vi "Reader.vi"() -> ()   [LabVIEW 2017]
uses:
  <vilib>/Instr/_visa.llb/VISA Configure Serial Port (Instr).vi
  <vilib>/picture/3D Picture Control/NI_3D Picture Control.lvlib
  <userlib>/_MGI/Numeric/Coercion/MGI Degrees to Radians/MGI Degrees to Radians DBL.vi
panel:
  out "result":i32
  out "sqrt(x)":dbl format="%#.1f"
  out "Samples (float)":dbl
  out "Gyro":cluster{"Pos X":dbl, "Pos Y":dbl, "Pos Z":dbl} {"Pos Z" format="%#.1f"; "Pos Y" format="%#.1f"; "Pos X" format="%#.1f"}
  out "Acc":cluster{"Pos X":dbl, "Pos Y":dbl, "Pos Z":dbl} {"Pos Z" format="%#.1f"; "Pos Y" format="%#.1f"; "Pos X" format="%#.1f"}
  out "Both":cluster{"Pos X":dbl, "Pos Y":dbl, "Pos Z":dbl} {"Pos Z" format="%#.1f"; "Pos Y" format="%#.1f"; "Pos X" format="%#.1f"}
  out "Pos":cluster{"Pos X":dbl, "Pos Y":dbl, "Pos Z":dbl} {"Pos Z" format="%#.1f"; "Pos Y" format="%#.1f"; "Pos X" format="%#.1f"}
  in  "Reading type":enum16{"ER_READ", "ER_BUF", "None"}(ring)
  in  "Fs reading":dbl=50.0 format="%#_13g"
  out "Acc Z":i16 caption="Z"
  out "Acc Y":i16 caption="Y"
  out "Acc X":i16 caption="X"
  out "Gyro Z":i16 caption="Z"
  out "Gyro Y":i16 caption="Y"
  out "Gyro X":i16 caption="X"
  out "Read":refnum<vi>(3d-picture)
  out "Samples (Int)":i32
  in  "Gyro LSB":dbl=131.0 format="%#_13g"
  out "error out":errorcluster
  out "Not recognized command":string
  in  "VISA resource name":refnum<visa-resource-name>="COM3"
  out "Gyro":refnum<vi>(3d-picture)
  out "Acc":refnum<vi>(3d-picture)
  in  "Gyro %":dbl=0.9 min=0.0 max=1.0 step=0.01
  out "Both":refnum<vi>(3d-picture)
  # "Comm setting"
  # "Positions"
  # "Reading"
  # "values"
  # "Acc"
  # "Gyro"
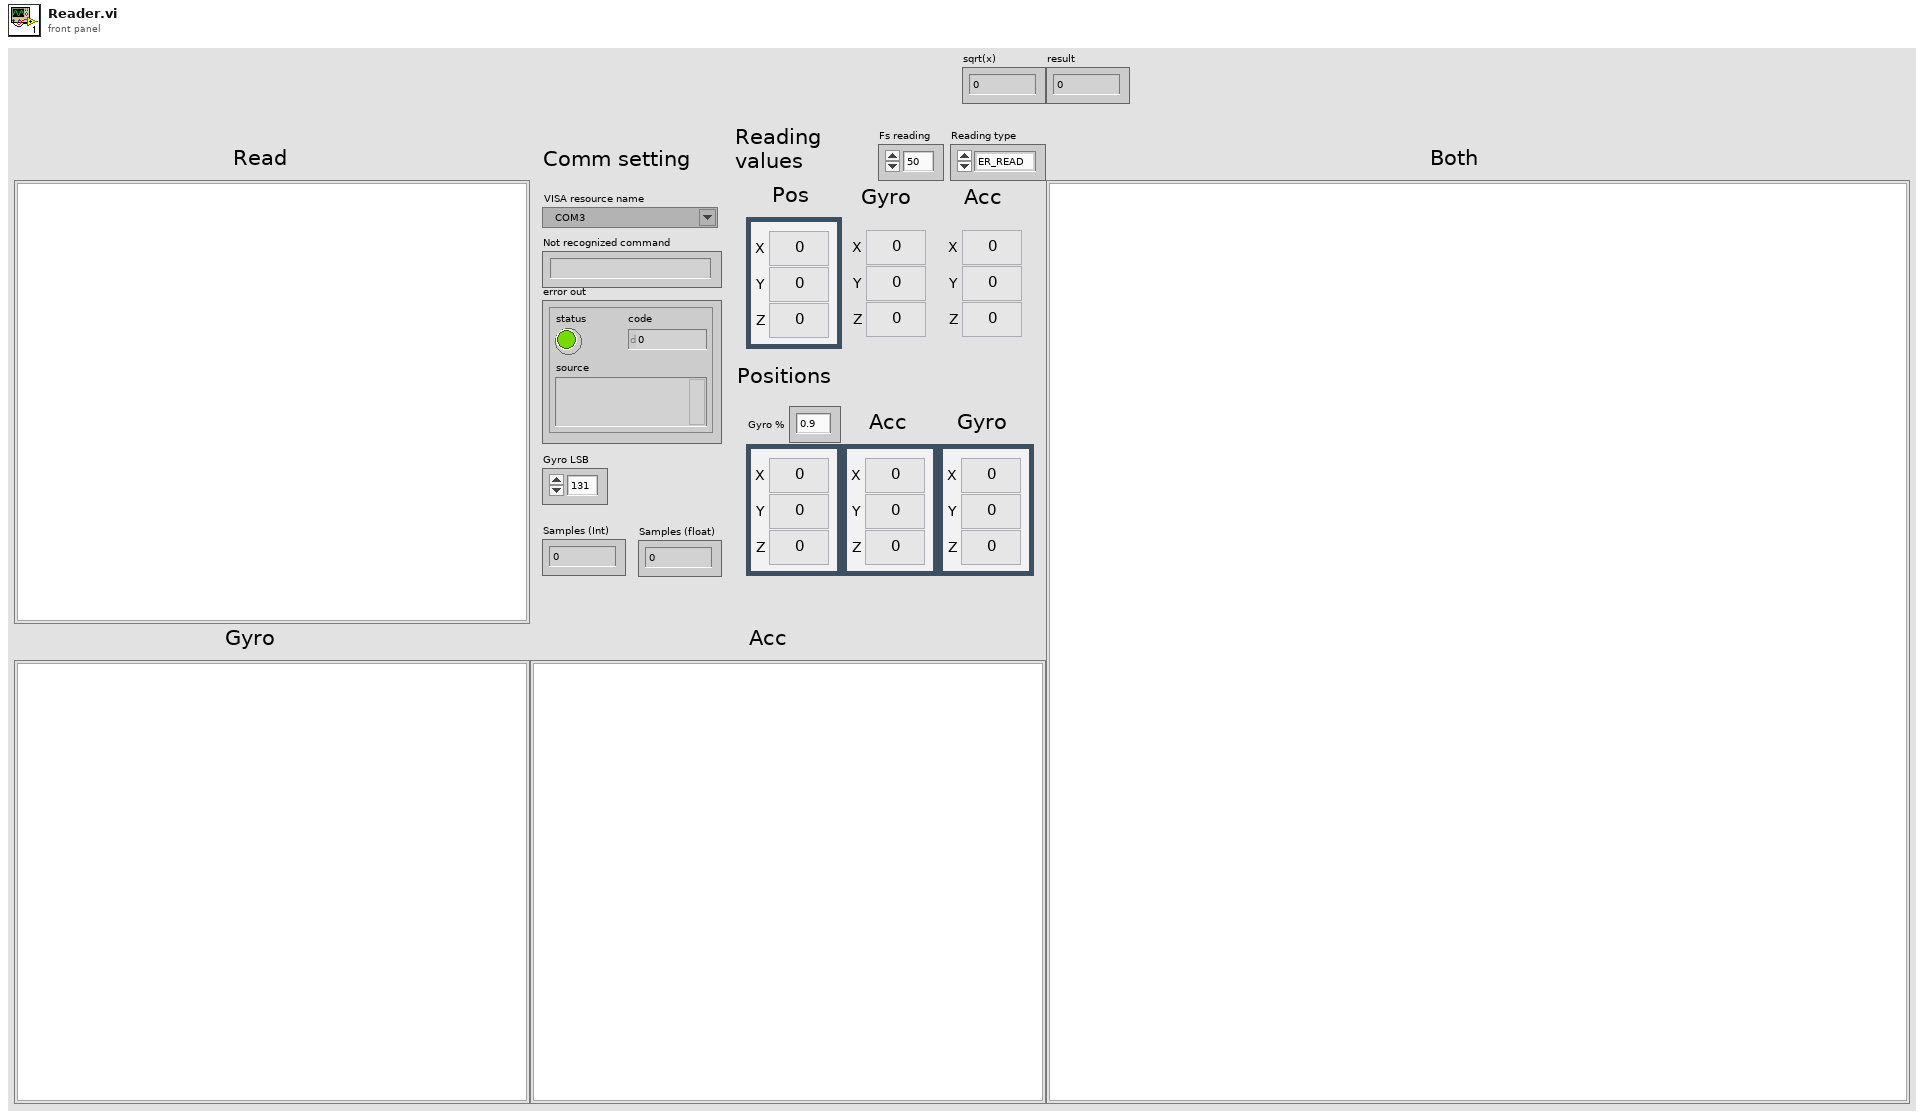
[diagram p1: front panel]
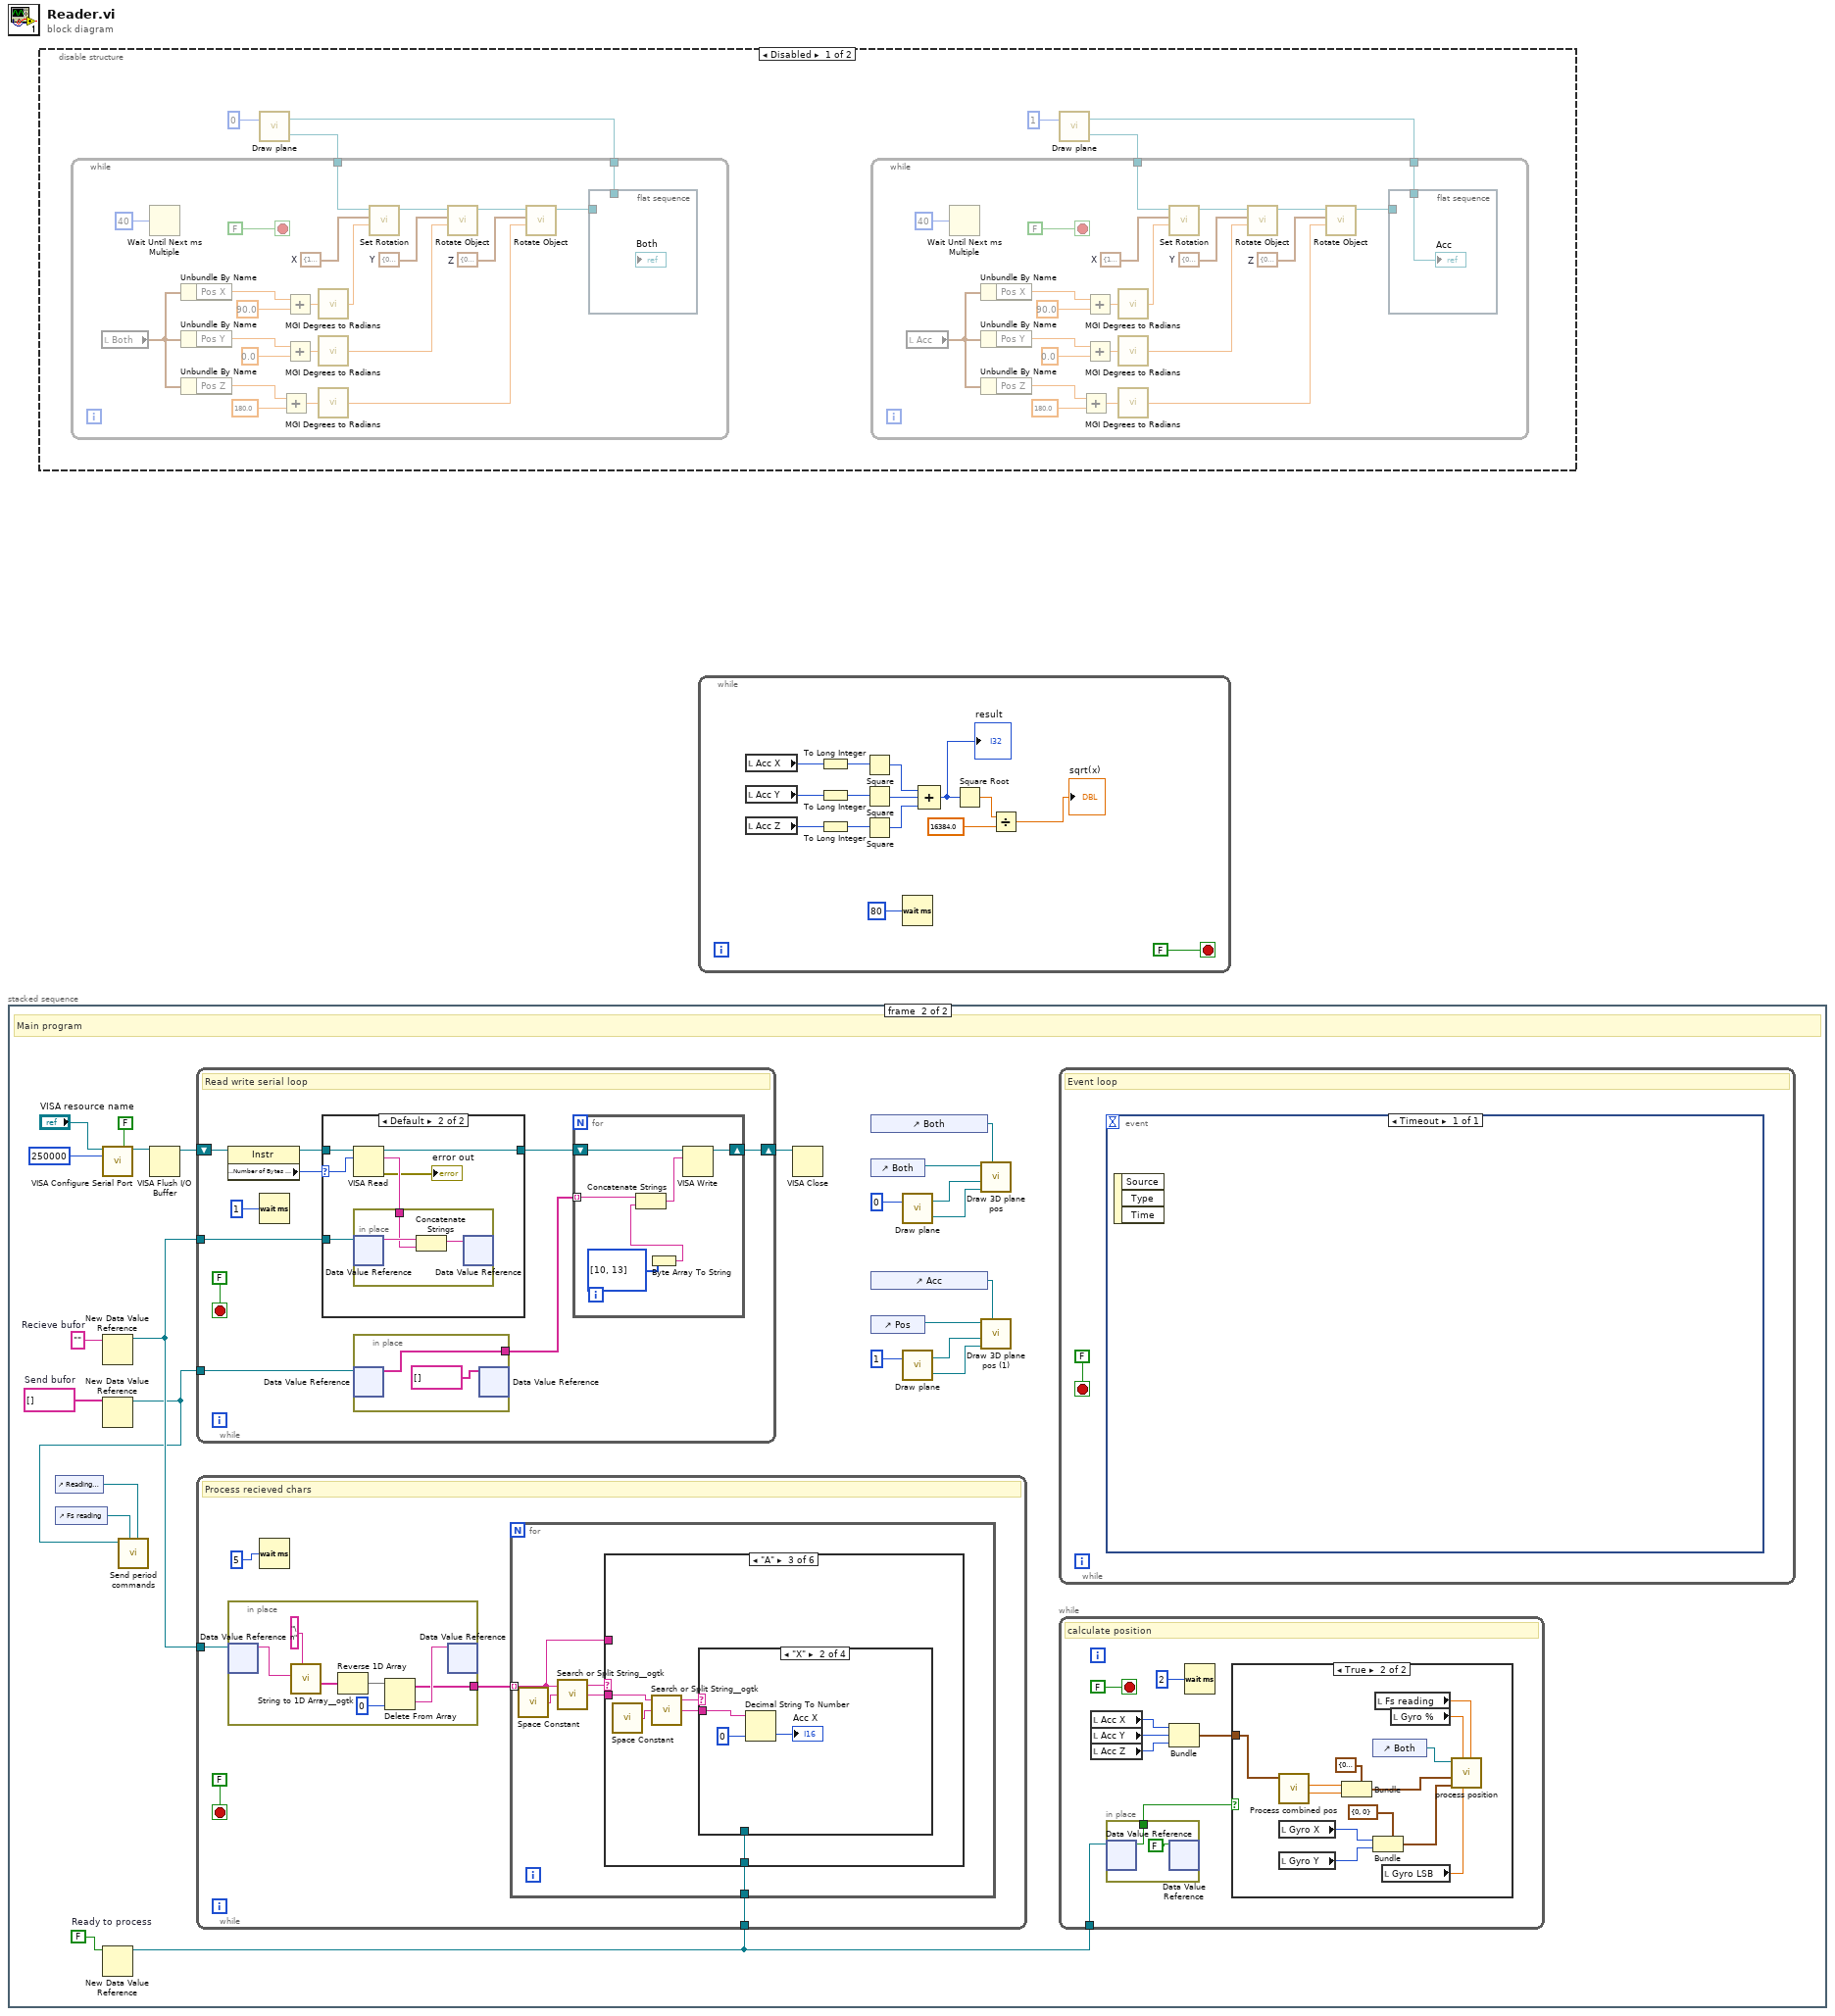
[diagram p0: block diagram]
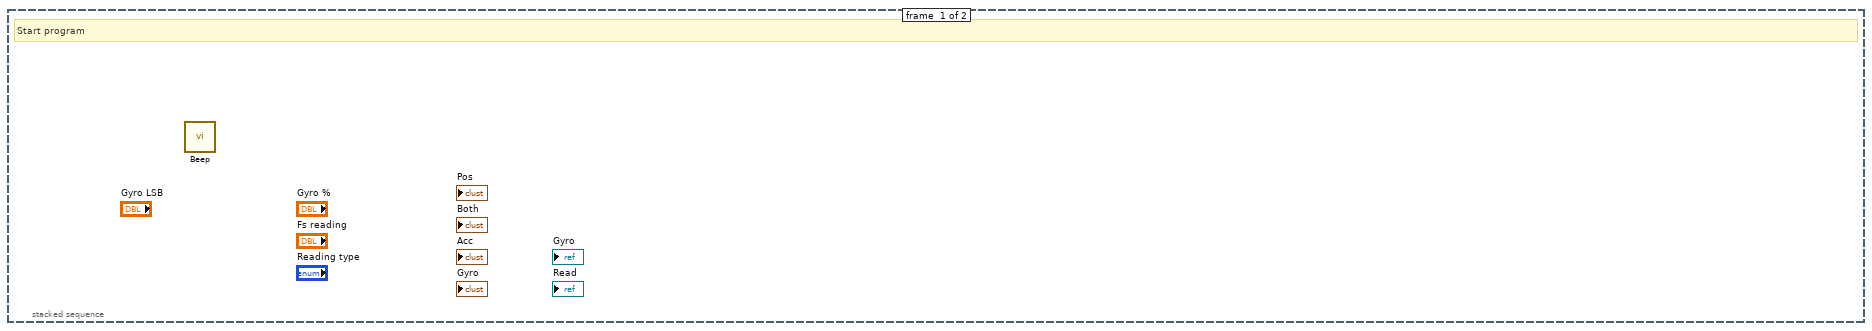
[diagram p3: hidden frame]
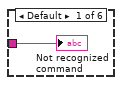
[diagram p5: hidden frame]
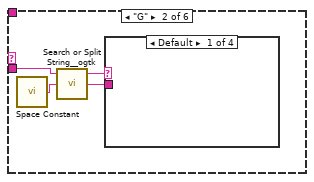
[diagram p6: hidden frame]
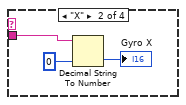
[diagram p7: hidden frame]
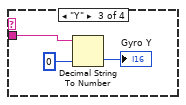
[diagram p8: hidden frame]
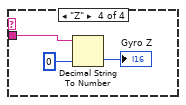
[diagram p9: hidden frame]
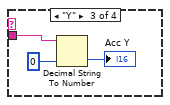
[diagram p11: hidden frame]
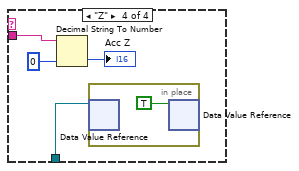
[diagram p12: hidden frame]
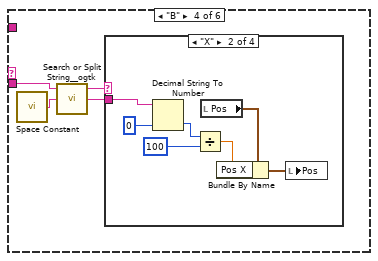
[diagram p13: hidden frame]
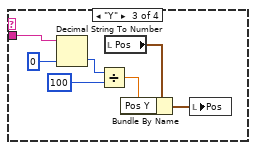
[diagram p15: hidden frame]
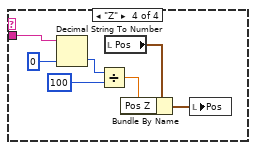
[diagram p16: hidden frame]
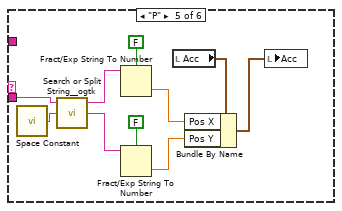
[diagram p17: hidden frame]
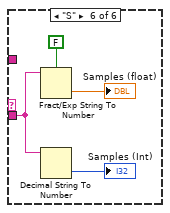
[diagram p18: hidden frame]
diagram:
  n1 = stacked-sequence {
    frame #0 {
      # "Start program"
      n2 = call <vilib>:"Beep.vi"() -> ()  [unwired: 12 in]
    }
    frame #1 {
      w15 = FALSE  # Ready to process
      w20 = string[] []  # Send bufor
      w21 = ""  # Recieve bufor
      # "Main program"
      n3 = control-ref of="Reading type"() -> (w11:refnum<vi>)
      n4 = control-ref of="Fs reading"() -> (w12:refnum<vi>)
      n5 = call-poly "VISA Configure Serial Port"("VISA resource name"="VISA resource name", "Enable Termination\nChar (T)"=FALSE ("Enable Termination\nChar (T)"), "baud rate (9600)"=u32 250000) -> ("VISA resource name out"=w17:refnum<visa-resource-name>)  [unwired: 11 in, 1 out]
      n6 = New Data Value Reference(data value=w21) -> (data value reference=w18:refnum<data-value>)  [unwired: 1 in, 1 out]
      n7 = New Data Value Reference(data value=w20) -> (data value reference=w13:refnum<data-value>)  [unwired: 1 in, 1 out]
      n8 = New Data Value Reference(data value=w15) -> (data value reference=w14:refnum<data-value>)  [unwired: 1 in, 1 out]
      n9 = call "Send period commands.vi"("Reading type ref"=w11, "Fs ref"=w12, "data value reference"=w13) -> ()  [unwired: 9 in]
      n10 = VISA Flush I/O Buffer(VISA resource name=w17) -> (VISA resource name out=w16:refnum<visa-resource-name>)  [unwired: 2 in, 1 out]
      n11 = while {
        tunnel: w18 -> [w140]
        shift-right: [w135] -> w19
        shift-left: w16 -> [w143]
        tunnel: w13 -> [w137]
        stop <- FALSE stop-if-true
        # "Read write serial loop"
        n12 = property class="Instr"(reference=w143) -> (reference out=w142:refnum<visa-resource-name>, "Serial Settings:Number of Bytes at Serial Port"=w141:u32)  [unwired: 1 in, 1 out]
        n13 = Wait (ms)(milliseconds to wait=u32 1) -> ()  [unwired: 1 out]
        n14 = case shown="Default" w141 {
          selector: w141 -> [_ w157]
          tunnel: w142 -> [w153 w158]
          tunnel: [w153 w156] -> w138
          tunnel: w140 -> [_ w159]
          frame 0 {
          }
          frame Default {
            n15 = VISA Read(VISA resource name=w158, byte count=w157) -> (VISA resource name out=w156:refnum<visa-resource-name>, read buffer=w155:string, error out=→"error out":errorcluster)  [unwired: 1 in, 1 out]
            n16 = in-place {
              in-place-border: w155 -> [w161]
              n17 = in-place-dvr #1(w159) -> (w162:string)  [unwired: 1 out]
              n18 = Concatenate Strings(w162, w161) -> (w160:string)
              n19 = in-place-dvr #1(w160) -> ()  [unwired: 2 out]
            }
          }
        }
        n20 = in-place {
          in-place-border: [w145] -> w136
          n21 = in-place-dvr #2(w137) -> (w145:string[])  [unwired: 1 out]
          n22 = in-place-dvr #2(string[] []) -> ()  [unwired: 2 out]
        }
        n23 = for {
          shift-right: [w151] -> w135
          shift-left: w138 -> [w152]
          tunnel: w136 -> [w150] mode=indexing
          n24 = Byte Array To String(unsigned byte array=u8[] [10, 13]) -> (string=w147:string)
          n25 = Concatenate Strings(w150, w147) -> (w149:string)
          n26 = VISA Write(VISA resource name=w152, write buffer=w149) -> (VISA resource name out=w151:refnum<visa-resource-name>)  [unwired: 1 in, 2 out]
        }
      }
      n27 = while {
        tunnel: w18 -> [w51]
        tunnel: w14 -> [w49]
        stop <- FALSE stop-if-true
        # "Process recieved chars"
        n28 = in-place {
          in-place-border: [w130] -> w50
          n29 = in-place-dvr #3(w51) -> (w134:string)  [unwired: 1 out]
          n30 = call <userlib>:"String to 1D Array__ogtk.vi"("delimiter (Tab)"="\n", "string"=w134) -> ("Array of Strings"=w129:string[])  [unwired: 9 in]
          n31 = Reverse 1D Array(array=w129) -> (reversed array=w128:string[])
          n32 = Delete From Array(array=w128, index=0) -> (deleted portion=w131:string, array with subset deleted=w130:string[])  [unwired: 1 in]
          n33 = in-place-dvr #3(w131) -> ()  [unwired: 2 out]
        }
        n34 = Wait (ms)(milliseconds to wait=u32 5) -> ()  [unwired: 1 out]
        n35 = for {
          tunnel: w50 -> [w54] mode=indexing
          tunnel: w49 -> [w55]
          n36 = call <vilib>:"Space Constant.vi"() -> ("String"=w58:string)
          n37 = call <userlib>:"Search or Split String__ogtk.vi"("search string/char (-)"=w58, "string"=w54) -> ("substring after match"=w56:string, "substring before match"=w57:string)  [unwired: 1 in, 1 out]
          n38 = case shown="\"A\"" w57 {
            tunnel: w56 -> [_ w62 w76 w91 w122 w126]
            tunnel: w54 -> [w59 _ _ _ _ _]
            tunnel: w55 -> [_ _ w73 _ _ _]
            frame Default {
              "Not recognized command" <- w59
            }
            frame "G" {
              n39 = call <vilib>:"Space Constant.vi"() -> ("String"=w63:string)
              n40 = call <userlib>:"Search or Split String__ogtk.vi"("search string/char (-)"=w63, "string"=w62) -> ("substring after match"=w60:string, "substring before match"=w61:string)  [unwired: 1 in, 1 out]
              n41 = case shown="Default" w61 {
                tunnel: w60 -> [_ w65 w67 w71]
                frame Default {
                }
                frame "X" {
                  n42 = Decimal String To Number(string=w65, default (0L)=i16 0 ("default (0 I32)")) -> (number=→"Gyro X":i16)  [unwired: 1 in, 1 out]
                }
                frame "Y" {
                  n43 = Decimal String To Number(string=w67, default (0L)=i16 0 ("default (0 I32)")) -> (number=→"Gyro Y":i16)  [unwired: 1 in, 1 out]
                }
                frame "Z" {
                  n44 = Decimal String To Number(string=w71, default (0L)=i16 0 ("default (0 I32)")) -> (number=→"Gyro Z":i16)  [unwired: 1 in, 1 out]
                }
              }
            }
            frame "A" {
              n45 = call <vilib>:"Space Constant.vi"() -> ("String"=w77:string)
              n46 = call <userlib>:"Search or Split String__ogtk.vi"("search string/char (-)"=w77, "string"=w76) -> ("substring after match"=w74:string, "substring before match"=w75:string)  [unwired: 1 in, 1 out]
              n47 = case shown="\"X\"" w75 {
                tunnel: w74 -> [_ w79 w82 w86]
                tunnel: w73 -> [_ _ _ w84]
                frame Default {
                }
                frame "X" {
                  n48 = Decimal String To Number(string=w79, default (0L)=i16 0 ("default (0 I32)")) -> (number=→"Acc X":i16)  [unwired: 1 in, 1 out]
                }
                frame "Y" {
                  n49 = Decimal String To Number(string=w82, default (0L)=i16 0 ("default (0 I32)")) -> (number=→"Acc Y":i16)  [unwired: 1 in, 1 out]
                }
                frame "Z" {
                  n50 = Decimal String To Number(string=w86, default (0L)=i16 0 ("default (0 I32)")) -> (number=→"Acc Z":i16)  [unwired: 1 in, 1 out]
                  n51 = in-place {
                    n52 = in-place-dvr #4(w84) -> ()  [unwired: 2 out]
                    n53 = in-place-dvr #4(TRUE ("data value")) -> ()  [unwired: 2 out]
                  }
                }
              }
            }
            frame "B" {
              n54 = call <vilib>:"Space Constant.vi"() -> ("String"=w92:string)
              n55 = call <userlib>:"Search or Split String__ogtk.vi"("search string/char (-)"=w92, "string"=w91) -> ("substring after match"=w89:string, "substring before match"=w90:string)  [unwired: 1 in, 1 out]
              n56 = case shown="\"X\"" w90 {
                tunnel: w89 -> [_ w98 w105 w112]
                frame Default {
                }
                frame "X" {
                  n57 = Decimal String To Number(string=w98, default (0L)=i16 0 ("default (0 I32)")) -> (number=w96:i16)  [unwired: 1 in, 1 out]
                  n58 = Divide(x=w96, y=i16 100) -> (x/y=w94:dbl)
                  n59 = local read "Pos"() -> (w95:cluster{"Pos X":dbl, "Pos Y":dbl, "Pos Z":dbl})
                  n60 = Bundle By Name(cluster=w95, "Pos X"=w94) -> (w93:cluster{"Pos X":dbl, "Pos Y":dbl, "Pos Z":dbl})
                  n61 = local write "Pos"(w93) -> ()
                }
                frame "Y" {
                  n62 = Decimal String To Number(string=w105, default (0L)=i16 0 ("default (0 I32)")) -> (number=w104:i16)  [unwired: 1 in, 1 out]
                  n63 = Divide(x=w104, y=i16 100) -> (x/y=w100:dbl)
                  n64 = local read "Pos"() -> (w102:cluster{"Pos X":dbl, "Pos Y":dbl, "Pos Z":dbl})
                  n65 = Bundle By Name(cluster=w102, "Pos Y"=w100) -> (w101:cluster{"Pos X":dbl, "Pos Y":dbl, "Pos Z":dbl})
                  n66 = local write "Pos"(w101) -> ()
                }
                frame "Z" {
                  n67 = Decimal String To Number(string=w112, default (0L)=i16 0 ("default (0 I32)")) -> (number=w111:i16)  [unwired: 1 in, 1 out]
                  n68 = Divide(x=w111, y=i16 100) -> (x/y=w107:dbl)
                  n69 = local read "Pos"() -> (w109:cluster{"Pos X":dbl, "Pos Y":dbl, "Pos Z":dbl})
                  n70 = Bundle By Name(cluster=w109, "Pos Z"=w107) -> (w108:cluster{"Pos X":dbl, "Pos Y":dbl, "Pos Z":dbl})
                  n71 = local write "Pos"(w108) -> ()
                }
              }
            }
            frame "P" {
              n72 = call <vilib>:"Space Constant.vi"() -> ("String"=w123:string)
              n73 = call <userlib>:"Search or Split String__ogtk.vi"("search string/char (-)"=w123, "string"=w122) -> ("substring after match"=w121:string, "substring before match"=w120:string)  [unwired: 1 in, 1 out]
              n74 = Fract/Exp String To Number(use system decimal point (T)=FALSE, string=w120) -> (number=w118:dbl)  [unwired: 2 in, 1 out]
              n75 = Fract/Exp String To Number(use system decimal point (T)=FALSE, string=w121) -> (number=w117:dbl)  [unwired: 2 in, 1 out]
              n76 = local read "Acc"() -> (w119:cluster{"Pos X":dbl, "Pos Y":dbl, "Pos Z":dbl})
              n77 = Bundle By Name(cluster=w119, "Pos X"=w118, "Pos Y"=w117) -> (w116:cluster{"Pos X":dbl, "Pos Y":dbl, "Pos Z":dbl})
              n78 = local write "Acc"(w116) -> ()
            }
            frame "S" {
              n79 = Fract/Exp String To Number(use system decimal point (T)=FALSE, string=w126) -> (number=→"Samples (float)":dbl)  [unwired: 2 in, 1 out]
              n80 = Decimal String To Number(string=w126) -> (number=→"Samples (Int)":i32)  [unwired: 2 in, 1 out]
            }
          }
        }
      }
      n81 = VISA Close(VISA resource name=w19) -> ()  [unwired: 1 in, 1 out]
      n82 = control-ref of="Both"() -> (w9:refnum<vi>)
      n83 = control-ref of="Both"() -> (w8:refnum<vi>)
      n84 = control-ref of="Acc"() -> (w4:refnum<vi>)
      n85 = control-ref of="Pos"() -> (w1:refnum<vi>)
      n86 = call "Draw plane.vi"("Number (0)"=u8 0) -> ("Modify object"=w7:refnum<vi>, "Draw object"=w6:refnum<vi>)  [unwired: 1 in]
      n87 = call "Draw plane.vi"("Number (0)"=u8 1) -> ("Modify object"=w2:refnum<vi>, "Draw object"=w3:refnum<vi>)  [unwired: 1 in]
      n88 = call "Draw 3D plane pos.vi"("3D picture ref"=w9, "Modify object"=w7, "Draw object"=w6, "Pos cluster ref"=w8) -> ()  [unwired: 8 in]
      n89 = call "Draw 3D plane pos (1).vi"("3D picture ref"=w4, "Modify object"=w2, "Draw object"=w3, "Pos cluster ref"=w1) -> ()  [unwired: 8 in]
      n90 = while {
        stop <- FALSE stop-if-true
        # "Event loop"
        n91 = event shown="[0] Timeout" {
          selector: _ -> [_]
          dyn-events: _ -> [_]
          timeout: _ -> [_]
          event Timeout {
            n92 = event-data() -> ()  [unwired: 1 in, 3 out]
          }
        }
      }
      n93 = while {
        tunnel: w14 -> [w27]
        stop <- FALSE stop-if-true
        # "calculate position"
        n94 = local read "Acc X"() -> (w30:i16)
        n95 = local read "Acc Y"() -> (w29:i16)
        n96 = local read "Acc Z"() -> (w31:i16)
        n97 = in-place {
          in-place-border: [w34] -> w26
          n98 = in-place-dvr #5(w27) -> (w34:bool)  [unwired: 1 out]
          n99 = in-place-dvr #5(FALSE ("data value")) -> ()  [unwired: 2 out]
        }
        n100 = Bundle("Acc X"=w30, "Acc Y"=w29, "Acc Z"=w31) -> (w28:cluster{"Acc X":i16, "Acc Y":i16, "Acc Z":i16})  [unwired: 1 in]
        n101 = Wait (ms)(milliseconds to wait=u32 2) -> ()  [unwired: 1 out]
        n102 = case shown="True" w26 {
          tunnel: w28 -> [_ w48]
          frame False {
          }
          frame True {
            n103 = call "Process combined pos.vi"("Acc data"=w48) -> ("Y processed"=w45:dbl, "X processed"=w46:dbl)  [unwired: 7 in, 2 out]
            n104 = local read "Gyro X"() -> (w43:i16)
            n105 = local read "Gyro Y"() -> (w42:i16)
            n106 = Bundle(cluster=cluster{"X acc":dbl, "Y acc":dbl} {"X acc"=0.0, "Y acc"=0.0}, "X acc"=w46, "Y acc"=w45) -> (w40:cluster{"X acc":dbl, "Y acc":dbl})
            n107 = control-ref of="Both"() -> (w47:refnum<vi>)
            n108 = Bundle(cluster=cluster{"Gyro X LSB":i16, "Gyro Y LSB":i16} {"Gyro X LSB"=0, "Gyro Y LSB"=0}, "Gyro X LSB"=w43, "Gyro Y LSB"=w42) -> (w39:cluster{"Gyro X LSB":i16, "Gyro Y LSB":i16})
            n109 = local read "Fs reading"() -> (w37:dbl)
            n110 = local read "Gyro LSB"() -> (w36:dbl)
            n111 = local read "Gyro %"() -> (w38:dbl)
            n112 = call "process position.vi"("Fs reading"=w37, "Gyro LSB"=w36, "Gyro %"=w38, "Gyro data"=w39, "Acc pos"=w40, "Pos cluster ref"=w47) -> ()  [unwired: 6 in]
          }
        }
      }
    }
  }
  n113 = disable-structure shown="Disabled" {
    frame Disabled {
      n114 = call "Draw plane.vi"("Number (0)"=u8 0) -> ("Modify object"=w166:refnum<vi>, "Draw object"=w167:refnum<vi>)  [unwired: 1 in]
      n115 = while {
        tunnel: w166 -> [w212]
        tunnel: w167 -> [w211]
        stop <- FALSE stop-if-true
        w208 = cluster{"X":sgl, "Y":sgl, "Z":sgl} {"X"=0.0, "Y"=0.0, "Z"=1.0}  # Z
        w209 = cluster{"X":sgl, "Y":sgl, "Z":sgl} {"X"=0.0, "Y"=1.0, "Z"=0.0}  # Y
        w215 = cluster{"X":sgl, "Y":sgl, "Z":sgl} {"X"=1.0, "Y"=0.0, "Z"=0.0}  # X
        n116 = local read "Both"() -> (w193:cluster{"Pos X":dbl, "Pos Y":dbl, "Pos Z":dbl})
        n117 = Wait Until Next ms Multiple(millisecond multiple=u32 40 ("milliseconds to wait")) -> ()  [unwired: 1 out]
        n118 = Unbundle By Name(w193) -> ("Pos X"=w197:dbl)
        n119 = Unbundle By Name(w193) -> ("Pos Y"=w196:dbl)
        n120 = Unbundle By Name(w193) -> ("Pos Z"=w195:dbl)
        n121 = Add(x=w195, y=180.0) -> (x+y=w204:dbl)
        n122 = Add(x=w197, y=90.0) -> (x+y=w200:dbl)
        n123 = Add(x=w196, y=0.0) -> (x+y=w203:dbl)
        n124 = call-poly <userlib>:"MGI Degrees to Radians.vi"("Degrees"=w200) -> ("Radians"=w213:dbl)
        n125 = call-poly <userlib>:"MGI Degrees to Radians.vi"("Degrees"=w203) -> ("Radians"=w210:dbl)
        n126 = call-poly <userlib>:"MGI Degrees to Radians.vi"("Degrees"=w204) -> ("Radians"=w207:dbl)
        n127 = call <vilib>:"Set Rotation.vi"("Angle"=w213, "Axis"=w215, "Scene Object"=w212) -> ("Rotated Scene Object"=w206:refnum<vi>)  [unwired: 7 in, 1 out]
        n128 = call <vilib>:"Rotate Object.vi"("Angle"=w210, "Axis"=w209, "Scene.Object In"=w206) -> ("Scene.Object Out"=w205:refnum<vi>)  [unwired: 7 in, 1 out]
        n129 = call <vilib>:"Rotate Object.vi"("Angle"=w207, "Axis"=w208, "Scene.Object In"=w205) -> ("Scene.Object Out"=w198:refnum<vi>)  [unwired: 7 in, 1 out]
        n130 = flat-sequence {
          tunnel: w211 -> [_]
          tunnel: w198 -> [_]
          frame #0 {
          }
        }
      }
      n131 = call "Draw plane.vi"("Number (0)"=u8 1) -> ("Modify object"=w164:refnum<vi>, "Draw object"=w163:refnum<vi>)  [unwired: 1 in]
      n132 = while {
        tunnel: w164 -> [w188]
        tunnel: w163 -> [w187]
        stop <- FALSE stop-if-true
        w184 = cluster{"X":sgl, "Y":sgl, "Z":sgl} {"X"=0.0, "Y"=0.0, "Z"=1.0}  # Z
        w185 = cluster{"X":sgl, "Y":sgl, "Z":sgl} {"X"=0.0, "Y"=1.0, "Z"=0.0}  # Y
        w191 = cluster{"X":sgl, "Y":sgl, "Z":sgl} {"X"=1.0, "Y"=0.0, "Z"=0.0}  # X
        n133 = local read "Acc"() -> (w169:cluster{"Pos X":dbl, "Pos Y":dbl, "Pos Z":dbl})
        n134 = Wait Until Next ms Multiple(millisecond multiple=u32 40 ("milliseconds to wait")) -> ()  [unwired: 1 out]
        n135 = Unbundle By Name(w169) -> ("Pos X"=w173:dbl)
        n136 = Unbundle By Name(w169) -> ("Pos Y"=w172:dbl)
        n137 = Unbundle By Name(w169) -> ("Pos Z"=w171:dbl)
        n138 = Add(x=w171, y=180.0) -> (x+y=w180:dbl)
        n139 = Add(x=w173, y=90.0) -> (x+y=w176:dbl)
        n140 = Add(x=w172, y=0.0) -> (x+y=w179:dbl)
        n141 = call-poly <userlib>:"MGI Degrees to Radians.vi"("Degrees"=w176) -> ("Radians"=w189:dbl)
        n142 = call-poly <userlib>:"MGI Degrees to Radians.vi"("Degrees"=w179) -> ("Radians"=w186:dbl)
        n143 = call-poly <userlib>:"MGI Degrees to Radians.vi"("Degrees"=w180) -> ("Radians"=w183:dbl)
        n144 = call <vilib>:"Set Rotation.vi"("Angle"=w189, "Axis"=w191, "Scene Object"=w188) -> ("Rotated Scene Object"=w182:refnum<vi>)  [unwired: 7 in, 1 out]
        n145 = call <vilib>:"Rotate Object.vi"("Angle"=w186, "Axis"=w185, "Scene.Object In"=w182) -> ("Scene.Object Out"=w181:refnum<vi>)  [unwired: 7 in, 1 out]
        n146 = call <vilib>:"Rotate Object.vi"("Angle"=w183, "Axis"=w184, "Scene.Object In"=w181) -> ("Scene.Object Out"=w174:refnum<vi>)  [unwired: 7 in, 1 out]
        n147 = flat-sequence {
          tunnel: w187 -> [w192]
          tunnel: w174 -> [_]
          frame #0 {
            "Acc" <- w192
          }
        }
      }
    }
    frame Enabled {
    }
  }
  n148 = while {
    stop <- FALSE stop-if-true
    n149 = local read "Acc X"() -> (w224:i16)
    n150 = local read "Acc Y"() -> (w222:i16)
    n151 = local read "Acc Z"() -> (w219:i16)
    n152 = To Long Integer(number=w224) -> (32bit integer=w223:i32)
    n153 = To Long Integer(number=w222) -> (32bit integer=w221:i32)
    n154 = To Long Integer(number=w219) -> (32bit integer=w220:i32)
    n155 = Square(x=w223) -> (x^2=w229:i32)
    n156 = Square(x=w221) -> (x^2=w228:i32)
    n157 = Square(x=w220) -> (x^2=w227:i32)
    n158 = Wait (ms)(milliseconds to wait=u32 80) -> ()  [unwired: 1 out]
    n159 = Compound Arithmetic op=ADD(w229, w228, w227) -> (w226:i32)
    "result" <- w226
    n160 = Square Root(x=w226) -> (sqrt(x)=w218:dbl)
    n161 = Divide(x=w218, y=16384.0) -> (x/y=→"sqrt(x)":dbl)
  }
